vi "Set Softlimit.vi"(8 "error in (no error)":errorcluster, 9 "P_limit":dbl, 10 "N_limit":dbl, 11 "Motor in":refnum<class "Motor.lvclass">) -> (0 "error out":errorcluster, 3 "Motor out":refnum<class "Motor.lvclass">)   [LabVIEW 2016, in "Hardware.lvlib" / "Motor.lvlib" / "Motor.lvclass"]
uses:
  <userlib>/Common Components/Hardware/Motor/Motor/Motor.lvclass
  <userlib>/Common Components/Hardware/Motor/Motor/Motor.lvclass/Motor.ctl
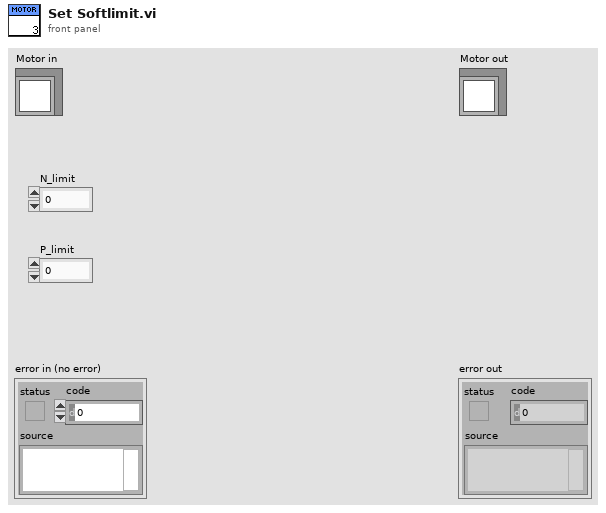
[diagram p1: front panel]
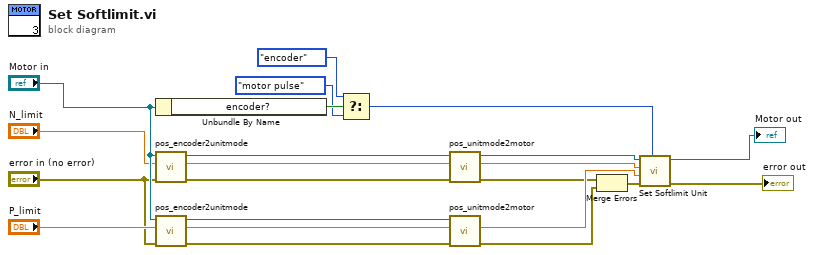
[diagram p0: block diagram]
diagram:
  n1 = Unbundle By Name("Motor in") -> ("encoder?"=w20:bool)
  n2 = call <userlib>:"pos_encoder2unitmode.vi"("error in (no error)"="error in (no error)", "encoder (unit)"="N_limit", "Motor in"="Motor in") -> ("error out"=w5:errorcluster, "pos in unit mode"=w12:dbl, "Motor out"=w16:refnum<class "Motor.lvclass">)  [unwired: 6 in]
  n3 = call <userlib>:"pos_encoder2unitmode.vi"("error in (no error)"="error in (no error)", "encoder (unit)"="P_limit", "Motor in"="Motor in") -> ("error out"=w6:errorcluster, "pos in unit mode"=w9:dbl, "Motor out"=w15:refnum<class "Motor.lvclass">)  [unwired: 6 in]
  n4 = Select(t=enum16{"motor pulse", "encoder"}."encoder" ("source_sel"), s=w20, f=enum16{"motor pulse", "encoder"}."motor pulse" ("source_sel")) -> (s? t:f=w19:enum16{"motor pulse", "encoder"})
  n5 = call <userlib>:"pos_unitmode2motor.vi"("error in (no error)"=w5, "pos in unit mode"=w12, "Motor in"=w16) -> ("error out"=w4:errorcluster, "pos in motor (pulses)"=w11:dbl, "Motor out"=w1:refnum<class "Motor.lvclass">)  [unwired: 6 in]
  n6 = call <userlib>:"pos_unitmode2motor.vi"("error in (no error)"=w6, "pos in unit mode"=w9, "Motor in"=w15) -> ("error out"=w3:errorcluster, "pos in motor (pulses)"=w8:dbl)  [unwired: 6 in, 1 out]
  n7 = Merge Errors(w4, w3) -> (w2:errorcluster)
  n8 = call-dynamic "Set Softlimit Unit.vi"("source_sel"=w19, "error in (no error)"=w2, "P_limit"=w8, "N_limit"=w11, "Motor in"=w1) -> ("error out"=→"error out":errorcluster, "Motor out"=→"Motor out":refnum<class "Motor.lvclass">)  [unwired: 5 in]
